vi "IR LED Final.vi"() -> ()   [LabVIEW 2023]
panel:
  out "IR Sensor":bool
  in  "stop":bool
  out "GREEN":bool
  out "Amber":bool
  out "RED":bool
  out "Counter":i32
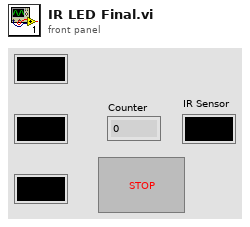
[diagram p1: front panel]
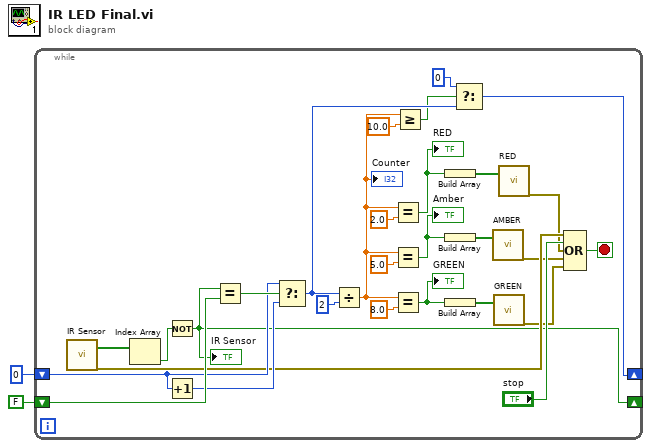
[diagram p0: block diagram]
diagram:
  n1 = while {
    shift-right: [w22] -> _
    shift-left: FALSE -> [w31]
    shift-right: [w5] -> _
    shift-left: 0 -> [w29]
    stop <- w25 stop-if-true
    n2 = call "IR Sensor"() -> ("data"=w27:bool[], "error out"=w24:errorcluster)  [unwired: 17 in, 1 out]
    n3 = Index Array(array=w27) -> (element=w26:bool)  [unwired: 1 in]
    n4 = Not(x=w26) -> (.not. x?=w22:bool)
    "IR Sensor" <- w22
    n5 = Increment(x=w29) -> (x+1=w28:i32)
    n6 = Equal?(x=w22, y=w31) -> (x = y?=w30:bool)
    n7 = Select(t=w29, s=w30, f=w28) -> (s? t:f=w6:i32)
    n8 = Divide(x=w6, y=2) -> (x/y=w8:dbl)
    "Counter" <- w8
    n9 = Equal?(x=w8, y=2.0) -> (x = y?=w15:bool)
    "RED" <- w15
    n10 = Equal?(x=w8, y=5.0) -> (x = y?=w13:bool)
    "Amber" <- w13
    n11 = Equal?(x=w8, y=8.0) -> (x = y?=w17:bool)
    "GREEN" <- w17
    n12 = Greater Or Equal?(x=w8, y=10.0) -> (x >= y?=w3:bool)
    n13 = Build Array(w15) -> (w14:bool[])
    n14 = Build Array(w13) -> (w12:bool[])
    n15 = Build Array(w17) -> (w16:bool[])
    n16 = Select(t=0, s=w3, f=w6) -> (s? t:f=w5:i32)
    n17 = call "AMBER"("data"=w12) -> ("error out"=w10:errorcluster)  [unwired: 17 in, 1 out]
    n18 = call "GREEN"("data"=w16) -> ("error out"=w9:errorcluster)  [unwired: 17 in, 1 out]
    n19 = call "RED"("data"=w14) -> ("error out"=w11:errorcluster)  [unwired: 17 in, 1 out]
    n20 = Compound Arithmetic op=OR(w24, "stop", w11, w10, w9) -> (w25:bool)
  }
